vi "WSVCAP SHL FPGA LL RFFE Read Data.vi"(11 "error in (no error)":errorcluster, 12 "Socket Mask":u64) -> (4 "Word Out (1-Bit for Each Channel)":u64, 15 "error out":errorcluster)   [LabVIEW 2017]
uses:
  <vilib>/eio/EIONode/EIONode.xnode
  WSVCAP SHL FPGA LL RFFE Debug Global.vi
  <vilib>/rvi/eio/common/nirviEmuTemplateMethod_errors.vi
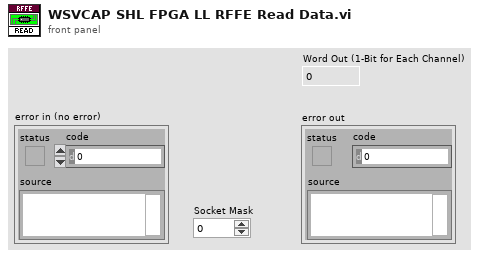
[diagram p1: front panel]
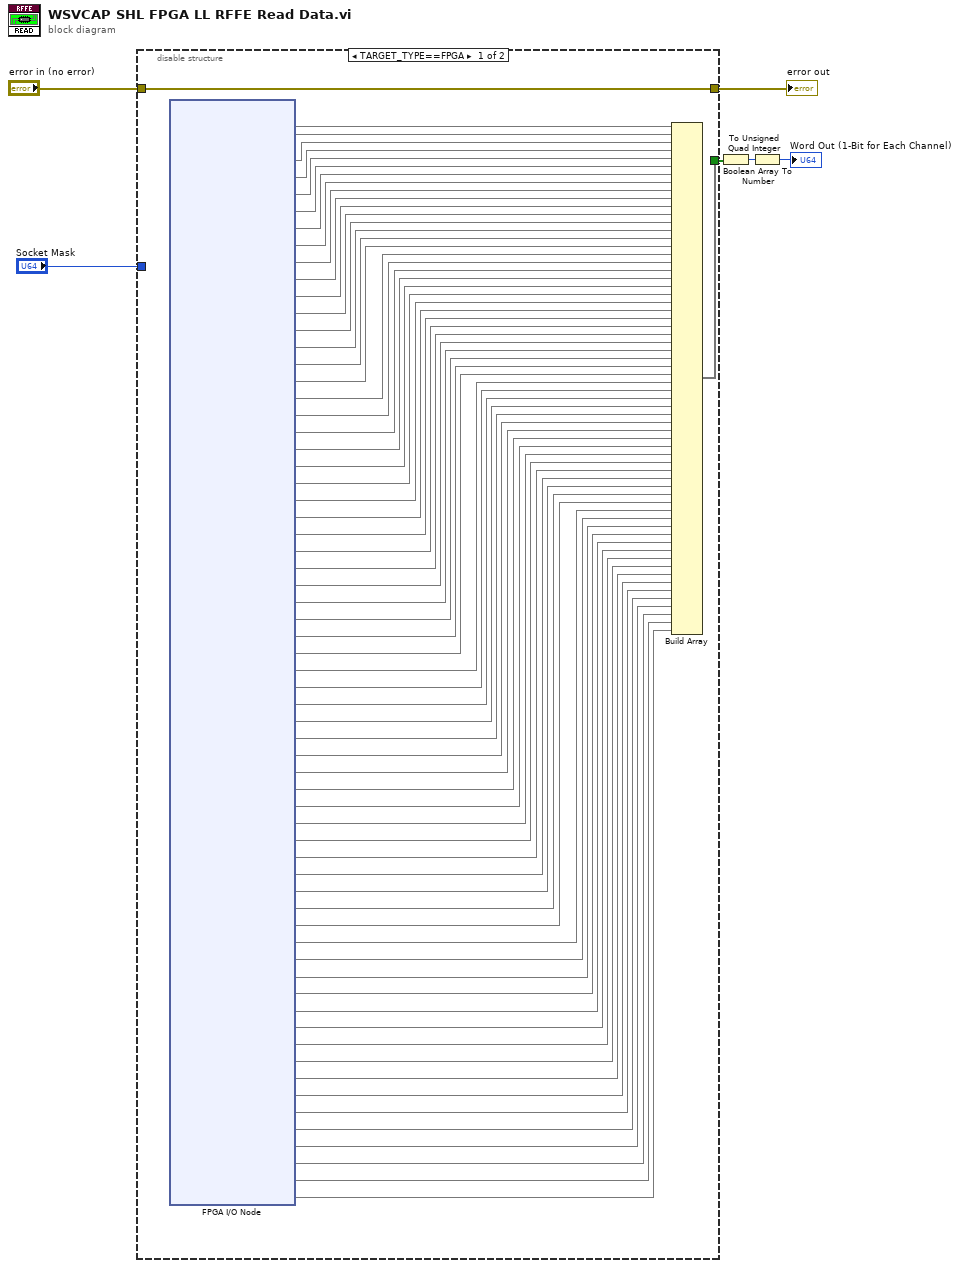
[diagram p0: block diagram]
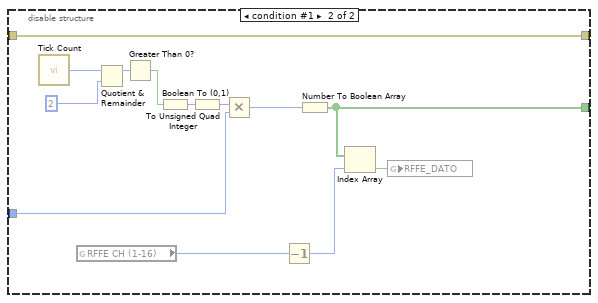
[diagram p2: hidden frame]
diagram:
  n1 = disable-structure shown="TARGET_TYPE==FPGA" {
    disable-tunnel: [w56 w75] -> w2
    disable-tunnel: [w55 w82] -> w6
    disable-tunnel: "error in (no error)" -> [w55 w82]
    disable-tunnel: "Socket Mask" -> [_ w79]
    frame condition #0 (active) {
      n2 = xnode "FPGA I/O Node"() -> ("RFFE_DATO_S1"=w57, "RFFE_DATO_S2"=w72, "RFFE_DATO_S3"=w71, "RFFE_DATO_S4"=w70, "RFFE_DATO_S5"=w69, "RFFE_DATO_S6"=w68, "RFFE_DATO_S7"=w67, "RFFE_DATO_S8"=w66, "RFFE_DATO_S9"=w65, "RFFE_DATO_S10"=w64, "RFFE_DATO_S11"=w63, "RFFE_DATO_S12"=w62, "RFFE_DATO_S13"=w61, "RFFE_DATO_S14"=w60, "RFFE_DATO_S15"=w59, "RFFE_DATO_S16"=w58, "RFFE_DATO_S17"=w54, "RFFE_DATO_S18"=w53, "RFFE_DATO_S19"=w52, "RFFE_DATO_S20"=w51, "RFFE_DATO_S21"=w50, "RFFE_DATO_S22"=w49, "RFFE_DATO_S23"=w48, "RFFE_DATO_S24"=w47, "RFFE_DATO_S25"=w46, "RFFE_DATO_S26"=w45, "RFFE_DATO_S27"=w44, "RFFE_DATO_S28"=w43, "RFFE_DATO_S29"=w42, "RFFE_DATO_S30"=w41, "RFFE_DATO_S31"=w40, "RFFE_DATO_S32"=w39, "RFFE_DATO_S33"=w38, "RFFE_DATO_S34"=w37, "RFFE_DATO_S35"=w36, "RFFE_DATO_S36"=w35, "RFFE_DATO_S37"=w34, "RFFE_DATO_S38"=w33, "RFFE_DATO_S39"=w32, "RFFE_DATO_S40"=w31, "RFFE_DATO_S41"=w30, "RFFE_DATO_S42"=w29, "RFFE_DATO_S43"=w28, "RFFE_DATO_S44"=w27, "RFFE_DATO_S45"=w26, "RFFE_DATO_S46"=w25, "RFFE_DATO_S47"=w24, "RFFE_DATO_S48"=w23, "RFFE_DATO_S49"=w22, "RFFE_DATO_S50"=w21, "RFFE_DATO_S51"=w20, "RFFE_DATO_S52"=w19, "RFFE_DATO_S53"=w18, "RFFE_DATO_S54"=w17, "RFFE_DATO_S55"=w16, "RFFE_DATO_S56"=w15, "RFFE_DATO_S57"=w14, "RFFE_DATO_S58"=w13, "RFFE_DATO_S59"=w12, "RFFE_DATO_S60"=w11, "RFFE_DATO_S61"=w10, "RFFE_DATO_S62"=w9, "RFFE_DATO_S63"=w8, "RFFE_DATO_S64"=w7)  [unwired: 64 in, 64 out]
      n3 = Build Array(w57, w72, w71, w70, w69, w68, w67, w66, w65, w64, w63, w62, w61, w60, w59, w58, w54, w53, w52, w51, w50, w49, w48, w47, w46, w45, w44, w43, w42, w41, w40, w39, w38, w37, w36, w35, w34, w33, w32, w31, w30, w29, w28, w27, w26, w25, w24, w23, w22, w21, w20, w19, w18, w17, w16, w15, w14, w13, w12, w11, w10, w9, w8, w7) -> (w56:void[])
    }
    frame condition #1 {
      n4 = call "Tick Count"() -> ("Tick Count(Ticks)"=w85:u32)
      n5 = global read "WSVCAP SHL FPGA LL RFFE Debug Global.vi" "RFFE CH (1-16)"() -> (w77:i32)
      n6 = Quotient & Remainder(x=w85, y=u32 2) -> (x-y*floor(x/y)=w84:u32)  [unwired: 1 out]
      n7 = Greater Than 0?(x=w84) -> (x > 0?=w73:bool)
      n8 = Boolean To (0,1)(Boolean=w73) -> (0, 1=w81:i16)
      n9 = To Unsigned Quad Integer(1:w81) -> (0:w80:u64)
      n10 = Multiply(x=w80, y=w79) -> (x*y=w78:u64)
      n11 = Decrement(x=w77) -> (x-1=w74:i32)
      n12 = Number To Boolean Array(number=w78) -> (Boolean array=w75:bool[])
      n13 = Index Array(array=w75, index=w74) -> (element=w76:bool)
      n14 = global write "WSVCAP SHL FPGA LL RFFE Debug Global.vi" "RFFE_DATO"(w76) -> ()
    }
  }
  "error out" <- w6
  n15 = Boolean Array To Number(Boolean array=w2) -> (number=w3:u64)
  n16 = To Unsigned Quad Integer(1:w3) -> (0:→"Word Out (1-Bit for Each Channel)":u64)
